vi "LINX - Analog Set Voltage Reference.vi"() -> ()   [LabVIEW 2019]
doc: "This example demonstrates how to set a LINX device's analog reference."
uses:
  <vilib>/MakerHub/LINX/Private/Device/Type Defs/AI Reference Mode.ctl
  <vilib>/MakerHub/LINX/Public/Peripherals/Analog/Analog Read 1 Chan.vi
  <vilib>/MakerHub/LINX/Public/Peripherals/Analog/Analog Read N Chans.vi
  <vilib>/MakerHub/LINX/Private/Local IO/LinxAnalogRead.vi
  <vilib>/MakerHub/LINX/Public/Utilities/Check Channel.vi
  <vilib>/MakerHub/LINX/Public/Utilities/Open Serial.vi
  <vilib>/MakerHub/LINX/Private/Utilties/Generate Error.vi
  <vilib>/MakerHub/LINX/LMH-LINX.lvlib
  <vilib>/MakerHub/LINX/Private/Device/Device.lvlib
panel:
  in  "Stop Button":bool
  in  "VISA resource name":refnum<visa-resource-name>
  out "AI Value":dbl
  in  "AI Reference Mode":T1
  in  "Analog Reference (V)":dbl=3.3
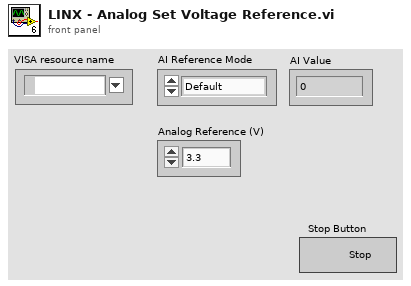
[diagram p1: front panel]
types:
  T1 = typedef "LMH-LINX.lvlib/Device.lvlib/AI Reference Mode.ctl" = enum16{"Default", "Internal", "External"}
  T2 = typedef "LMH-LINX.lvlib/LINX Ref.ctl" = cluster{"IO":T3, "Interface":T4, "LINX Device Config":T5}
  T3 = typedef "LMH-LINX.lvlib/Platform.ctl" = enum16{"Remote", "Local"}
  T4 = typedef "LMH-LINX.lvlib/Interface.ctl" = enum16{"Serial", "TCP"}
  T5 = typedef "LMH-LINX.lvlib/Device.lvlib/LINX Device Config.ctl" = cluster{"Interface":T4, "COM Port":refnum<visa-resource-name>, "TCP Configuration":T6, "Device Family":u8, "Device ID":u8, "Device Name":string, "TCP Ref":refnum<k5>, "Channels":T7}
  T6 = typedef "LMH-LINX.lvlib/Device.lvlib/TCP Config.ctl" = cluster{"IP Address":string, "Port":u16}
  T7 = typedef "LMH-LINX.lvlib/Channels.ctl" = cluster{"DI":u8[], "DO":u8[], "AI":u8[], "AO":u8[], "PWM":u8[], "QE":u8[], "UART":u8[], "I2C 2":u8[], "SPI":u8[], "CAN":u8[], "Servo":u8[], "AI Ref (V)":dbl, "AI Resolution (Bits)":u8, "AO Ref (V)":dbl, "AO Resolution (Bits)":u8}
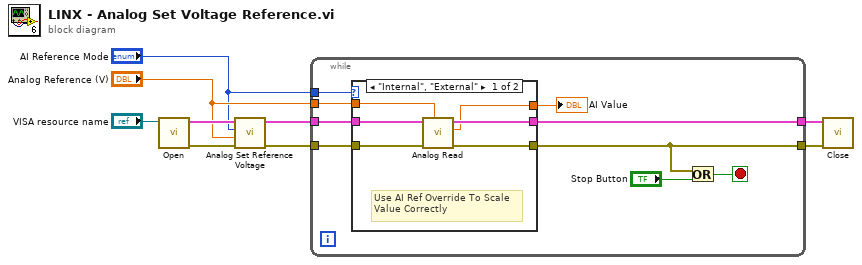
[diagram p0: block diagram]
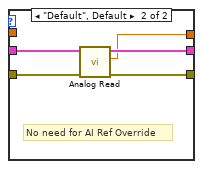
[diagram p2: hidden frame]
diagram:
  n1 = call-poly <vilib>:"Open.vi"("Serial Port"="VISA resource name") -> ("Error Out"=w8:errorcluster, "LINX Resource"=w9:T2)  [unwired: 8 in, 1 out]
  n2 = call <vilib>:"Analog Set Reference Voltage.vi"("Error In"=w8, "Analog Reference (V)"="Analog Reference (V)", "AI Reference Mode"="AI Reference Mode", "LINX Ref in"=w9) -> ("Error Out"=w7:errorcluster, "LINX Ref out"=w6:T2)  [unwired: 6 in]
  n3 = while {
    tunnel: w7 -> [w18]
    tunnel: w6 -> [w17]
    tunnel: [w12] -> w5
    tunnel: [w16] -> w4
    tunnel: "Analog Reference (V)" -> [w15]
    tunnel: "AI Reference Mode" -> [w10]
    stop <- w13 stop-if-true
    n4 = case shown="\"Internal\", \"External\"" w10 {
      tunnel: w18 -> [w24 w29]
      tunnel: w17 -> [w23 w28]
      tunnel: [w22 w27] -> w16
      tunnel: w15 -> [w21 _]
      tunnel: [w20 w26] -> w14
      tunnel: [w19 w25] -> w12
      frame "Internal", "External" {
        # "Use AI Ref Override To Scale\nValue Correctly"
        n5 = call-poly <vilib>:"Analog Read.vi"("Analog Ref Override (V)"=w21, "Error In"=w24, "LINX Resource"=w23) -> ("Error Out"=w19:errorcluster, "Voltage"=w20:dbl, "LINX Resource"=w22:T2)  [unwired: 5 in, 1 out]
      }
      frame "Default", Default {
        # "No need for AI Ref Override"
        n6 = call-poly <vilib>:"Analog Read.vi"("Error In"=w29, "LINX Resource"=w28) -> ("Error Out"=w25:errorcluster, "Voltage"=w26:dbl, "LINX Resource"=w27:T2)  [unwired: 6 in, 1 out]
      }
    }
    "AI Value" <- w14
    n7 = Or(x=w12, y="Stop Button") -> (x .or. y?=w13:bool)
  }
  n8 = call <vilib>:"Close.vi"("Error In"=w5, "LINX Resource"=w4) -> ()  [unwired: 9 in, 1 out]
